vi "Initialize Front Panel.vi"(8 "error in (no error)":errorcluster, 11 "Test Executive Builder Active Info View in":refnum<class "Test Executive Builder Active Info View.lvclass">) -> (0 "error out":errorcluster, 3 "Test Executive Builder Active Info View out":refnum<class "Test Executive Builder Active Info View.lvclass">)   [LabVIEW 2017, in "Test Executive Builder Active Info View.lvclass"]
doc: "<License>\nCopyright © 2017 Composed Systems, LLC | All rights reserved\nwww.composed.io\n\nAuthor: Ethan Stern <ethan.stern@composed.io>\n\nThis software is provided \"AS IS\" WITHOUT WARRANTIES, either express or implied, AND IS FOR EDUCATIONAL PURPOSES ONLY.\n</License>"
uses:
  Test Executive Builder Active Info View.lvclass
  <vilib>/gpm_packages/@cs/mva-viewable/Source/IViewManager/IViewManager/IViewManager.lvclass
  <vilib>/gpm_packages/@cs/mva-viewable/Source/IViewable/IViewable Messages/Insert Front Panel Msg/Insert Front Panel Msg.lvclass
  C:/Users/jonmc/Documents/Git/Test Executive Builder/gpm_packages/@cs/mva-framework/Source/Framework/IViewManager/IViewManager/IViewManager.lvclass
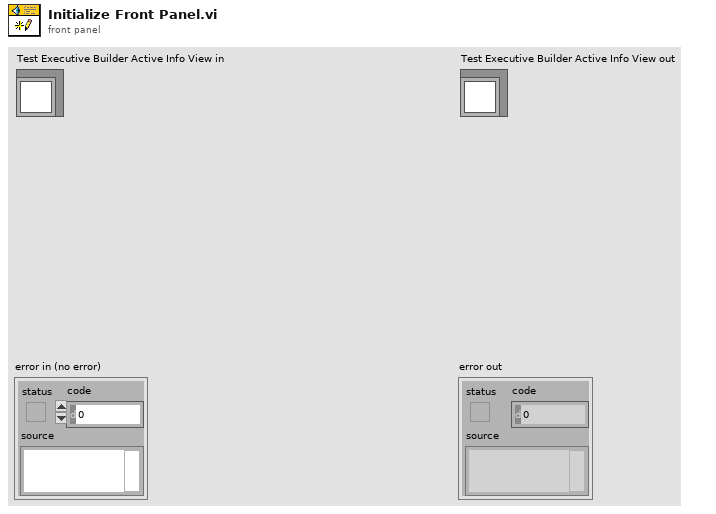
[diagram p1: front panel]
types:
  T1 = typedef "IViewable.lvlib/ProtectedSubpanel.lvclass/Protected Subpanel Reference.ctl" = refnum<data-value>
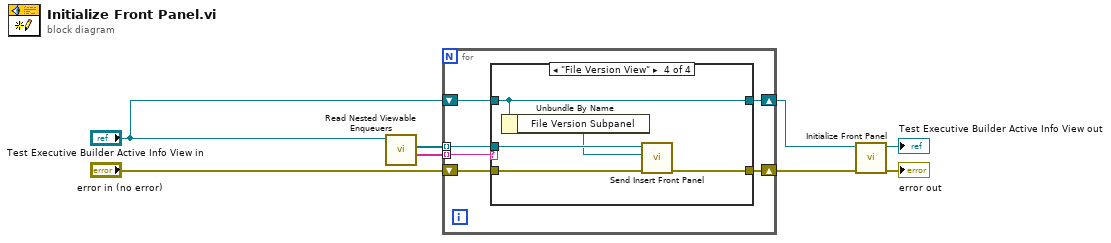
[diagram p0: block diagram]
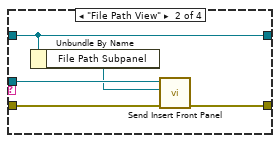
[diagram p3: hidden frame]
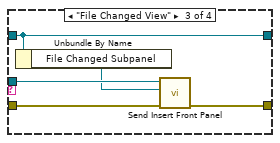
[diagram p4: hidden frame]
diagram:
  n1 = call <vilib>:"Read Nested Viewable Enqueuers.vi"("IViewManager in"="Test Executive Builder Active Info View in") -> ("Viewable Names"=w6:string[], "Nested Viewable Enqueuers"=w5:refnum<class "Message Enqueuer.lvclass">[])  [unwired: 9 in]
  n2 = for {
    tunnel: w6 -> [w10] mode=indexing
    tunnel: w5 -> [w14] mode=indexing
    shift-right: [w12] -> w3
    shift-left: "error in (no error)" -> [w13]
    shift-right: [w9] -> w1
    shift-left: "Test Executive Builder Active Info View in" -> [w11]
    n3 = case shown="\"File Version View\"" w10 {
      tunnel: w14 -> [_ w21 w26 w31]
      tunnel: w13 -> [w15 w19 w24 w29]
      tunnel: [w15 w18 w23 w28] -> w12
      tunnel: w11 -> [w16 w17 w22 w27]
      tunnel: [w16 w17 w22 w27] -> w9
      frame Default {
      }
      frame "File Path View" {
        n4 = Unbundle By Name(w17) -> ("File Path Subpanel"=w20:T1)
        n5 = call <vilib>:"Send Insert Front Panel.vi"("error in (no error)"=w19, "Protected Subpanel"=w20, "Message Enqueuer"=w21) -> ("error out"=w18:errorcluster)  [unwired: 7 in, 1 out]
      }
      frame "File Changed View" {
        n6 = Unbundle By Name(w22) -> ("File Changed Subpanel"=w25:T1)
        n7 = call <vilib>:"Send Insert Front Panel.vi"("error in (no error)"=w24, "Protected Subpanel"=w25, "Message Enqueuer"=w26) -> ("error out"=w23:errorcluster)  [unwired: 7 in, 1 out]
      }
      frame "File Version View" {
        n8 = Unbundle By Name(w27) -> ("File Version Subpanel"=w30:T1)
        n9 = call <vilib>:"Send Insert Front Panel.vi"("error in (no error)"=w29, "Protected Subpanel"=w30, "Message Enqueuer"=w31) -> ("error out"=w28:errorcluster)  [unwired: 7 in, 1 out]
      }
    }
  }
  n10 = call-parent "Initialize Front Panel.vi"("error in (no error)"=w3, "IViewable in"=w1) -> ("error out"=→"error out":errorcluster, "IViewable out"=→"Test Executive Builder Active Info View out":refnum<class "Test Executive Builder Active Info View.lvclass">)  [unwired: 8 in]
